vi "Control_Calibration.vi"(10 "Calibrated":bool, 11 "Raw Oculus Data":T2) -> (3 "Control":T1)   [LabVIEW 2017]
uses:
  Raw Oculus Data.ctl
  Calibration Control.ctl
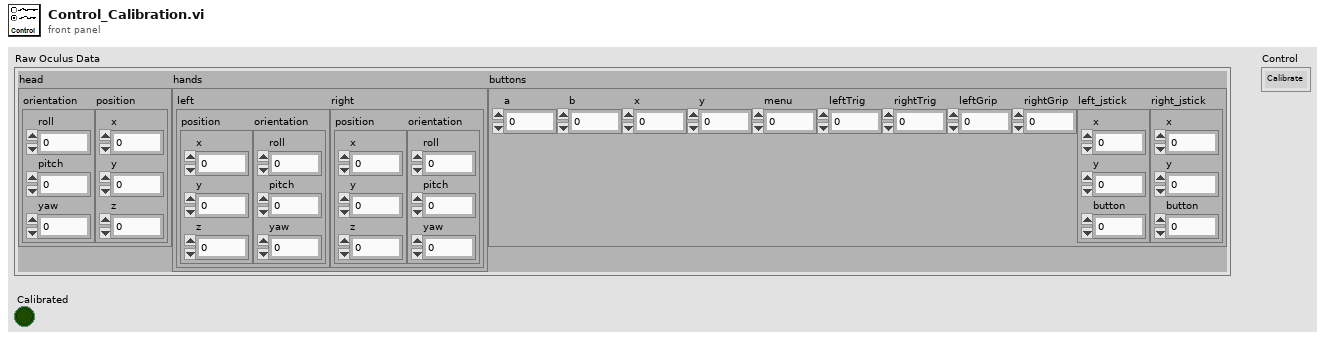
[diagram p1: front panel]
types:
  T1 = typedef "Calibration Control.ctl" = enum16{"Calibrate", "Max", "Min"}
  T2 = typedef "Raw Oculus Data.ctl" = cluster{"head":cluster{"orientation":cluster{"roll":dbl, "pitch":dbl, "yaw":dbl}, "position":cluster{"x":dbl, "y":dbl, "z":dbl}}, "hands":cluster{"left":cluster{"position":cluster{"x":dbl, "y":dbl, "z":dbl}, "orientation":cluster{"roll":dbl, "pitch":dbl, "yaw":dbl}}, "right":cluster{"position":cluster{"x":dbl, "y":dbl, "z":dbl}, "orientation":cluster{"roll":dbl, "pitch":dbl, "yaw":dbl}}}, "buttons":cluster{"a":i32, "b":i32, "x":i32, "y":i32, "menu":i32, "leftTrig":dbl, "rightTrig":dbl, "leftGrip":dbl, "rightGrip":dbl, "left_jstick":cluster{"x":dbl, "y":dbl, "button":i32}, "right_jstick":cluster{"x":dbl, "y":dbl, "button":i32}}}
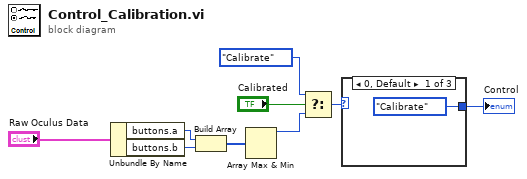
[diagram p0: block diagram]
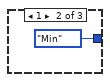
[diagram p2: hidden frame]
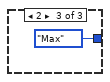
[diagram p3: hidden frame]
diagram:
  n1 = Unbundle By Name("Raw Oculus Data") -> ("buttons.a"=w2:i32, "buttons.b"=w3:i32)
  n2 = Build Array(w2, w3) -> (w1:i32[])
  n3 = Array Max & Min(array=w1) -> (max value=w9:i32)  [unwired: 3 out]
  n4 = Select(t=Calibration_Control."Calibrate" ("Control"), s="Calibrated", f=w9) -> (s? t:f=w8:i32)
  n5 = case shown="0, Default" w8 {
    tunnel: [Calibration_Control."Calibrate" ("Control") Calibration_Control."Min" ("Control") Calibration_Control."Max" ("Control")] -> w4
    frame 0, Default {
    }
    frame 1 {
    }
    frame 2 {
    }
  }
  "Control" <- w4
